vi "Test_Seq.vi"(8 "error in (no error)":errorcluster, 11 "Input":bool) -> (0 "error out":errorcluster, 3 "PASS?":bool)   [LabVIEW 2023]
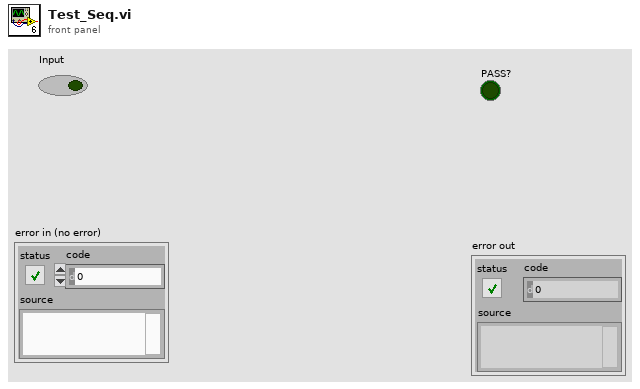
[diagram p1: front panel]
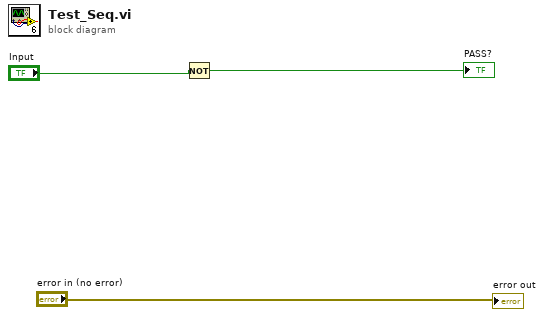
[diagram p0: block diagram]
diagram:
  n1 = Not(x="Input") -> (.not. x?=→"PASS?":bool)
  "error out" <- "error in (no error)"
